vi "Get Connections - 1Pin 1 Conn.vi"(6 "pin type":T1, 8 "error in":errorcluster, 9 "site":i32=-1, 10 "pin or relay name":string, 11 "session reservation in":refnum<class "Session Reservation.lvclass">) -> (0 "error out":errorcluster, 2 "connection":T2, 3 "session reservation out":refnum<class "Session Reservation.lvclass">)   [LabVIEW 2025, in "Session Management daqmxDI.lvlib"]
uses:
  Session Management daqmxDI.lvlib
  <vilib>/Plug-In SDKs/Clients/Session Management V1/Session Reservation/Session Reservation.lvclass
  Connection with Session.ctl
  <vilib>/Plug-In SDKs/Clients/Session Management V1/Session Reservation/Connection.ctl
  <vilib>/Plug-In SDKs/Clients/Session Management V1/Session Reservation/Pin Type.ctl
  Session Factory/Session Factory.lvclass
  fa653d4d-6a17-425d-94c9-d5d80778c854.vi
  fa653d4d-6a17-425d-94c9-d5d80778c854.vi/d089b476-b30c-4b91-b2ff-fbae0086b065.vi
  <vilib>/Plug-In SDKs/Clients/Session Management V1/Session Reservation/Pin to Pin Array.vi
  <vilib>/Plug-In SDKs/Clients/Session Management V1/Session Reservation/Get Connections Impl.vi
  <vilib>/Plug-In SDKs/Measurements/Helpers/Error Strings Global Internal.vi
  <vilib>/Utility/error.llb/Error Cluster From Error Code.vi
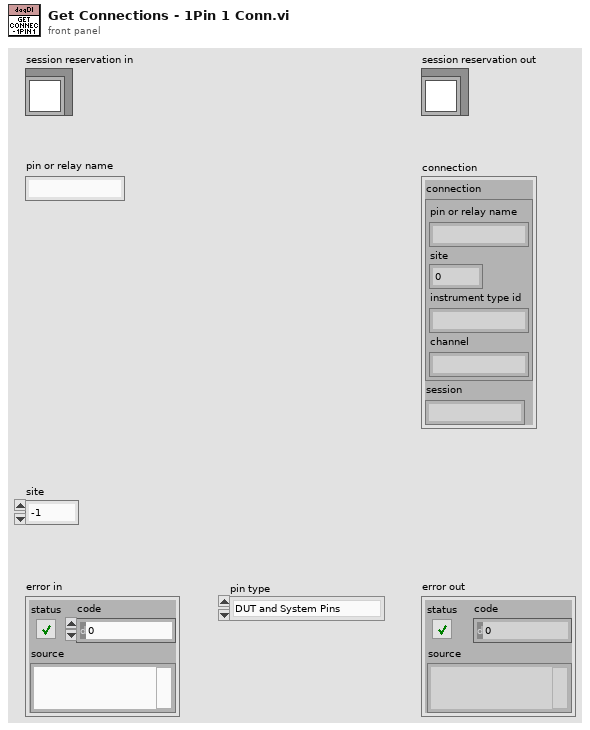
[diagram p1: front panel]
types:
  T1 = typedef "NI Session Management V1 Client.lvlib/Session Reservation.lvclass/Pin Type.ctl" = enum16{"DUT and System Pins", "System Pins"}
  T2 = typedef "Session Management daqmxDI.lvlib/Connection with Session.ctl" = cluster{"connection":T3, "session":string}
  T3 = typedef "NI Session Management V1 Client.lvlib/Session Reservation.lvclass/Connection.ctl" = cluster{"pin or relay name":string, "site":i32, "instrument type id":string, "channel":string}
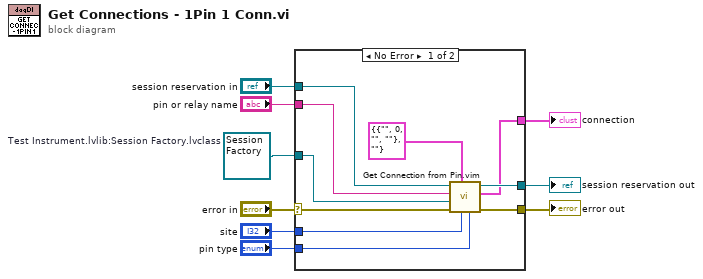
[diagram p0: block diagram]
diagram:
  w2 = refnum<class "Session Factory.lvclass"> refnum  # Test Instrument.lvlib:Session Factory.lvclass
  n1 = case shown="No Error" "error in" {
    selector: "error in" -> [w13 w20]
    tunnel: "session reservation in" -> [w19 w21]
    tunnel: "pin or relay name" -> [w14 _]
    tunnel: [w18 w20] -> w6
    tunnel: [w17 w21] -> w5
    tunnel: "site" -> [w12 _]
    tunnel: "pin type" -> [w11 _]
    tunnel: w2 -> [w10 _]
    tunnel: [w15 _] -> w1
    frame No Error {
      n2 = call "Get Connection from Pin.vim"("pin type"=w11, "site"=w12, "connection type"=T2 {"connection"={"pin or relay name"="", "site"=0, "instrument type id"="", "channel"=""}, "session"=""} ("connection with session"), "error in"=w13, "session factory"=w10, "pin or relay name"=w14, "session reservation in"=w19) -> ("error out"=w18:errorcluster, "connection"=w15:T2, "session reservation out"=w17:refnum<class "Session Reservation.lvclass">)  [unwired: 2 in]
    }
    frame Error {
    }
  }
  "error out" <- w6
  "session reservation out" <- w5
  "connection" <- w1
